vi "XY Graph Get Plot & Scale Arrays.vi"(8 "error in":errorcluster, 10 "Scale Labels in":string[](array[string]), 11 "Plot Names in":string[](array[string])) -> (0 "error out":errorcluster, 1 "Alternating Axes?":bool, 2 "Plot Scales Array":T1(array[cluster]), 3 "Plot Names Array":string[](array[string]))   [LabVIEW 2019]
uses:
  <vilib>/Utility/error.llb/Error Cluster From Error Code.vi
  <vilib>/ErrorRing/Error Ring.xnode
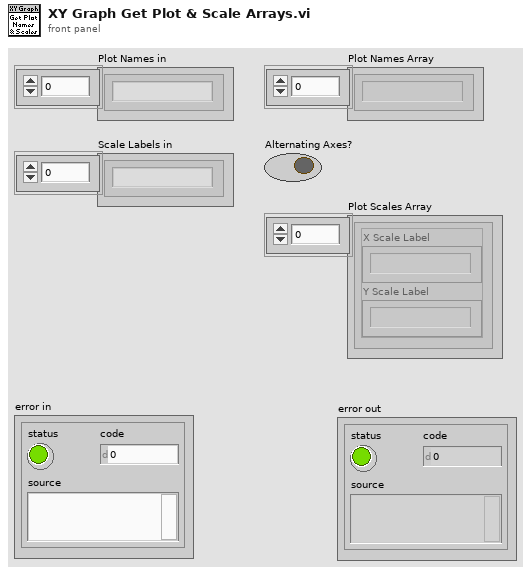
[diagram p1: front panel]
types:
  T1 = cluster{"X Scale Label":string, "Y Scale Label":string}[]
  T2 = cluster{"Scale Label":string, "Scale Label":string}
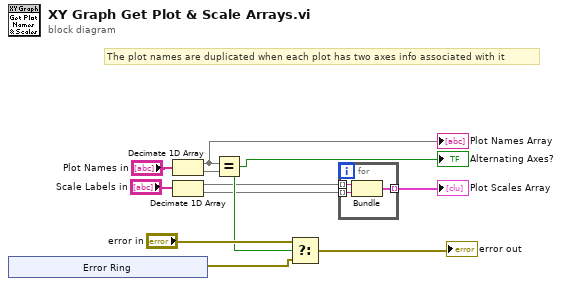
[diagram p0: block diagram]
diagram:
  # "The plot names are duplicated when each plot has two axes info associated with it"
  n1 = xnode "Error Ring"() -> ("error out"=w1:errorcluster)
  n2 = Decimate 1D Array("Plot Names in") -> (w4:string[], w3:string[])
  "Plot Names Array" <- w4
  n3 = Decimate 1D Array("Scale Labels in") -> (w6:string[], w7:string[])
  n4 = Equal?(x=w4, y=w3) -> (x = y?=w9:bool)
  "Alternating Axes?" <- w9
  n5 = Select(t="error in", s=w9, f=w1) -> (s? t:f=→"error out":errorcluster)
  n6 = for {
    tunnel: w6 -> [w14] mode=indexing
    tunnel: w7 -> [w13] mode=indexing
    tunnel: [w12] -> w8 mode=indexing
    n7 = Bundle("Scale Label"=w14, "Scale Label"=w13) -> (w12:T2)  [unwired: 1 in]
  }
  "Plot Scales Array" <- w8
